vi "Make Channels Coincident.vi"(6 "interp. method":i32(ring) items=["nearest", "linear", "spline", "cubic Hermite", "Lagrange"], 8 "Time Cluster 2":T1, 9 "Time Cluster 1":T1, 10 "Cluster 2":T2={"Colour"=0, "Inst type"=enum."Pitot-static tube", "Inst name"="Manometer voltage", "Symbol"="U", "Code name"="", "Extra Info"="U", "Inst Array"=enum."PWA", "Extra Titles"=[], "Extra Values"=[], "U"=0.0, "u^2"=0.0, "u^3"=0.0, "u^4"=0.0, "Skew_u"=0.0, "Kurt_u"=0.0, "Sd Error in Mean"=0.0, "% u'/U"=0.0, "X"=0.0, "Y"=0.0, "Z"=0.0, "Timescale integral Estimate"=0.0, "Sd Error in Variance"=0.0, "Calib File"=path "", "Calib Constants"=[], "Output Position"=FALSE, "Stats"=enum."None", "Av Sampling Rate"=0.0, "Av No of Samples"=0.0, "Total Meas Time (s)"=0.0, "ADAM Ch Name"="", "Max value"=0.0, "Min value"=0.0, "Req Sample Rate Hz"=0.0, "Sync Delay Time (s)"=0.0, "Ch No"=0, "Device"="", "Use Latest Calib"=FALSE, "Port"="", "Metadata Ch Names"=[], "Metadata Ch Values"=[], "Label"=""} {"Sync Delay Time (s)" format="%.4f"; "Total Meas Time (s)" format="%_5g"; "Sd Error in Variance" format="%_3g"; "Skew_u" format="%_3g"; "% u'/U" format="%_3g"; "Sd Error in Mean" format="%_3g"; "Kurt_u" format="%_3g"; "u^4" format="%_3g"; "u^3" format="%_3g"; "U" format="%_3g"; "u^2" format="%_3g"}, 11 "Cluster 1":T2={"Colour"=0, "Inst type"=enum."Pitot-static tube", "Inst name"="Manometer voltage", "Symbol"="U", "Code name"="", "Extra Info"="U", "Inst Array"=enum."PWA", "Extra Titles"=[], "Extra Values"=[], "U"=0.0, "u^2"=0.0, "u^3"=0.0, "u^4"=0.0, "Skew_u"=0.0, "Kurt_u"=0.0, "Sd Error in Mean"=0.0, "% u'/U"=0.0, "X"=0.0, "Y"=0.0, "Z"=0.0, "Timescale integral Estimate"=0.0, "Sd Error in Variance"=0.0, "Calib File"=path "", "Calib Constants"=[], "Output Position"=FALSE, "Stats"=enum."None", "Av Sampling Rate"=0.0, "Av No of Samples"=0.0, "Total Meas Time (s)"=0.0, "ADAM Ch Name"="", "Max value"=0.0, "Min value"=0.0, "Req Sample Rate Hz"=0.0, "Sync Delay Time (s)"=0.0, "Ch No"=0, "Device"="", "Use Latest Calib"=FALSE, "Port"="", "Metadata Ch Names"=[], "Metadata Ch Values"=[], "Label"=""} {"Sync Delay Time (s)" format="%.4f"; "Total Meas Time (s)" format="%_5g"; "Sd Error in Variance" format="%_3g"; "Skew_u" format="%_3g"; "% u'/U" format="%_3g"; "Sd Error in Mean" format="%_3g"; "Kurt_u" format="%_3g"; "u^4" format="%_3g"; "u^3" format="%_3g"; "U" format="%_3g"; "u^2" format="%_3g"}) -> (0 "Time Window (ms)":dbl, 1 "Coincident Time Cluster 2":T1, 3 "Coincident Time Cluster 1":T1)   [LabVIEW 2021]
uses:
  Controls/Inst_type.ctl
  Controls/Instrument_Array.ctl
  Controls/Analysis_info_cluster.ctl
  Controls/Time_Trace_Cluster.ctl
panel:
  out "Time Window (ms) 2":dbl
  out "Array":i32[](array[numeric])
  out "Boolean":bool
  out "Frame":string
  in  "Show Plots":bool
  out "U1 and U2 Raw":cluster{"yi":dbl[], "yi":dbl[]}[](graph)
  out "U1 and U2 made coincident":cluster{"yi":dbl[], "yi":dbl[]}[](graph)
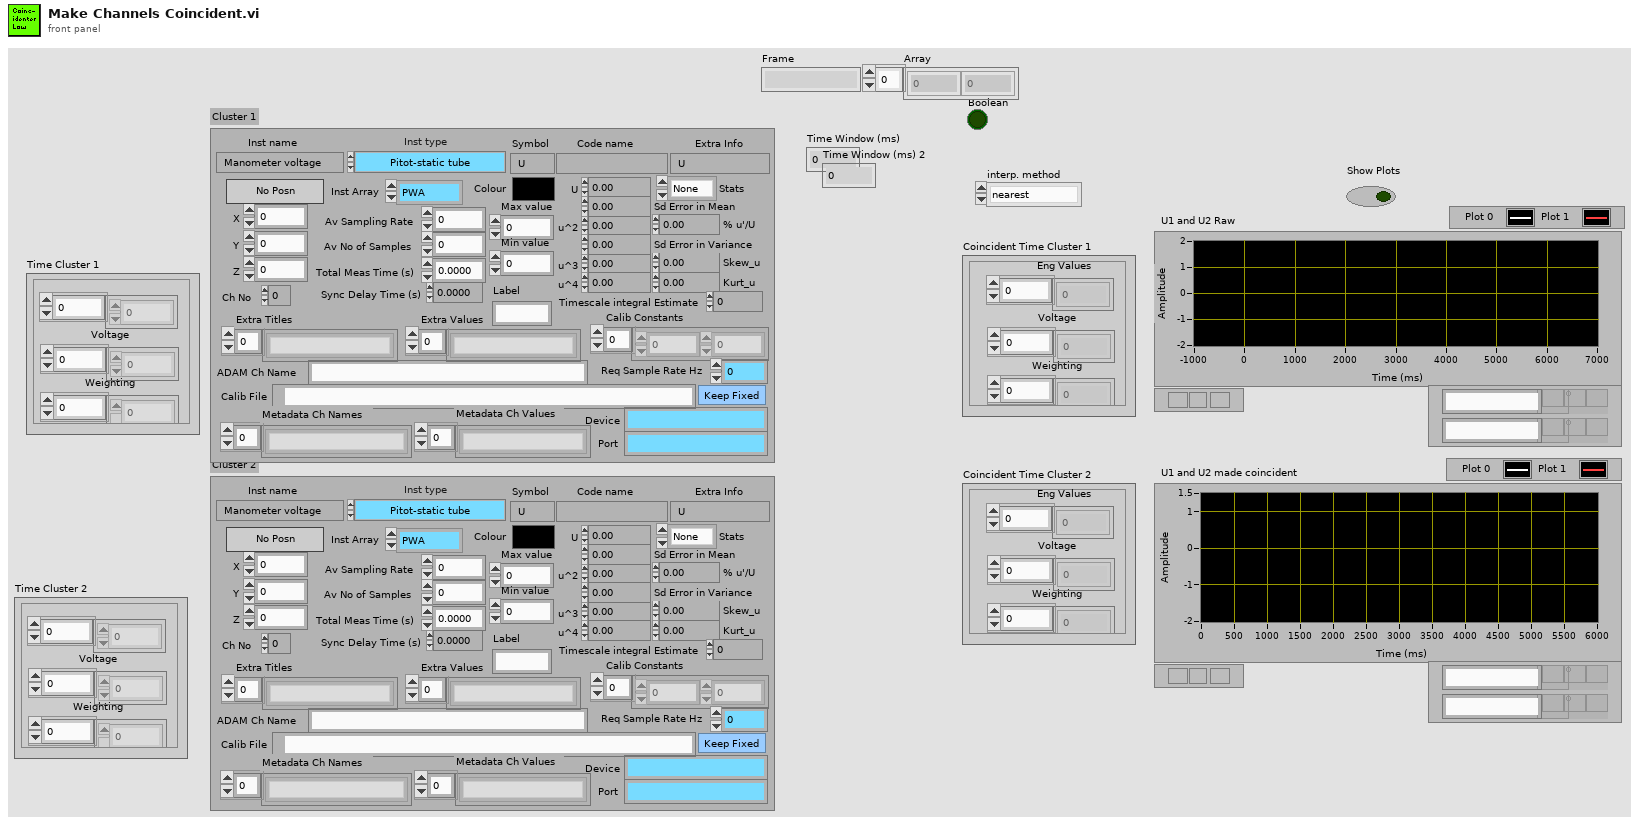
[diagram p1: front panel]
types:
  T1 = typedef "Time_Trace_Cluster.ctl" = cluster{"Weighting":dbl[], "Voltage":dbl[], "Eng Values":dbl[]}
  T2 = typedef "Analysis_info_cluster.ctl" = cluster{"Colour":u32, "Inst type":T3, "Inst name":string, "Symbol":string, "Code name":string, "Extra Info":string, "Inst Array":T4, "Extra Titles":string[], "Extra Values":string[], "U":dbl, "u^2":dbl, "u^3":dbl, "u^4":dbl, "Skew_u":dbl, "Kurt_u":dbl, "Sd Error in Mean":dbl, "% u'/U":dbl, "X":dbl, "Y":dbl, "Z":dbl, "Timescale integral Estimate":dbl, "Sd Error in Variance":dbl, "Calib File":path, "Calib Constants":dbl[], "Output Position":bool, "Stats":enum16{"None", "Basic", "Full"}, "Av Sampling Rate":dbl, "Av No of Samples":dbl, "Total Meas Time (s)":dbl, "ADAM Ch Name":string, "Max value":dbl, "Min value":dbl, "Req Sample Rate Hz":dbl, "Sync Delay Time (s)":dbl, "Ch No":i16, "Device":string, "Use Latest Calib":bool, "Port":string, "Metadata Ch Names":string[], "Metadata Ch Values":string[], "Label":string}
  T3 = typedef "Inst_type.ctl" = enum16{"Raw voltage", "Raw with zero offsetting", "Propeller anemometer", "Pressure Transducer", "Pitot-static tube", "Hot wire", "Cross wire 1", "Cross wire 2", "Generic Linear", "Generic Polynomial", "Generic BackPoly", "Fast FID", "Thermocouple", "Cold wire", "Pulsed Wire", "LDA Vel", "LDA Tran time", "LDA Arr time", "Microphone"}
  T4 = typedef "Instrument_Array.ctl" = enum16{"PWA", "LDA", "Analogue"}
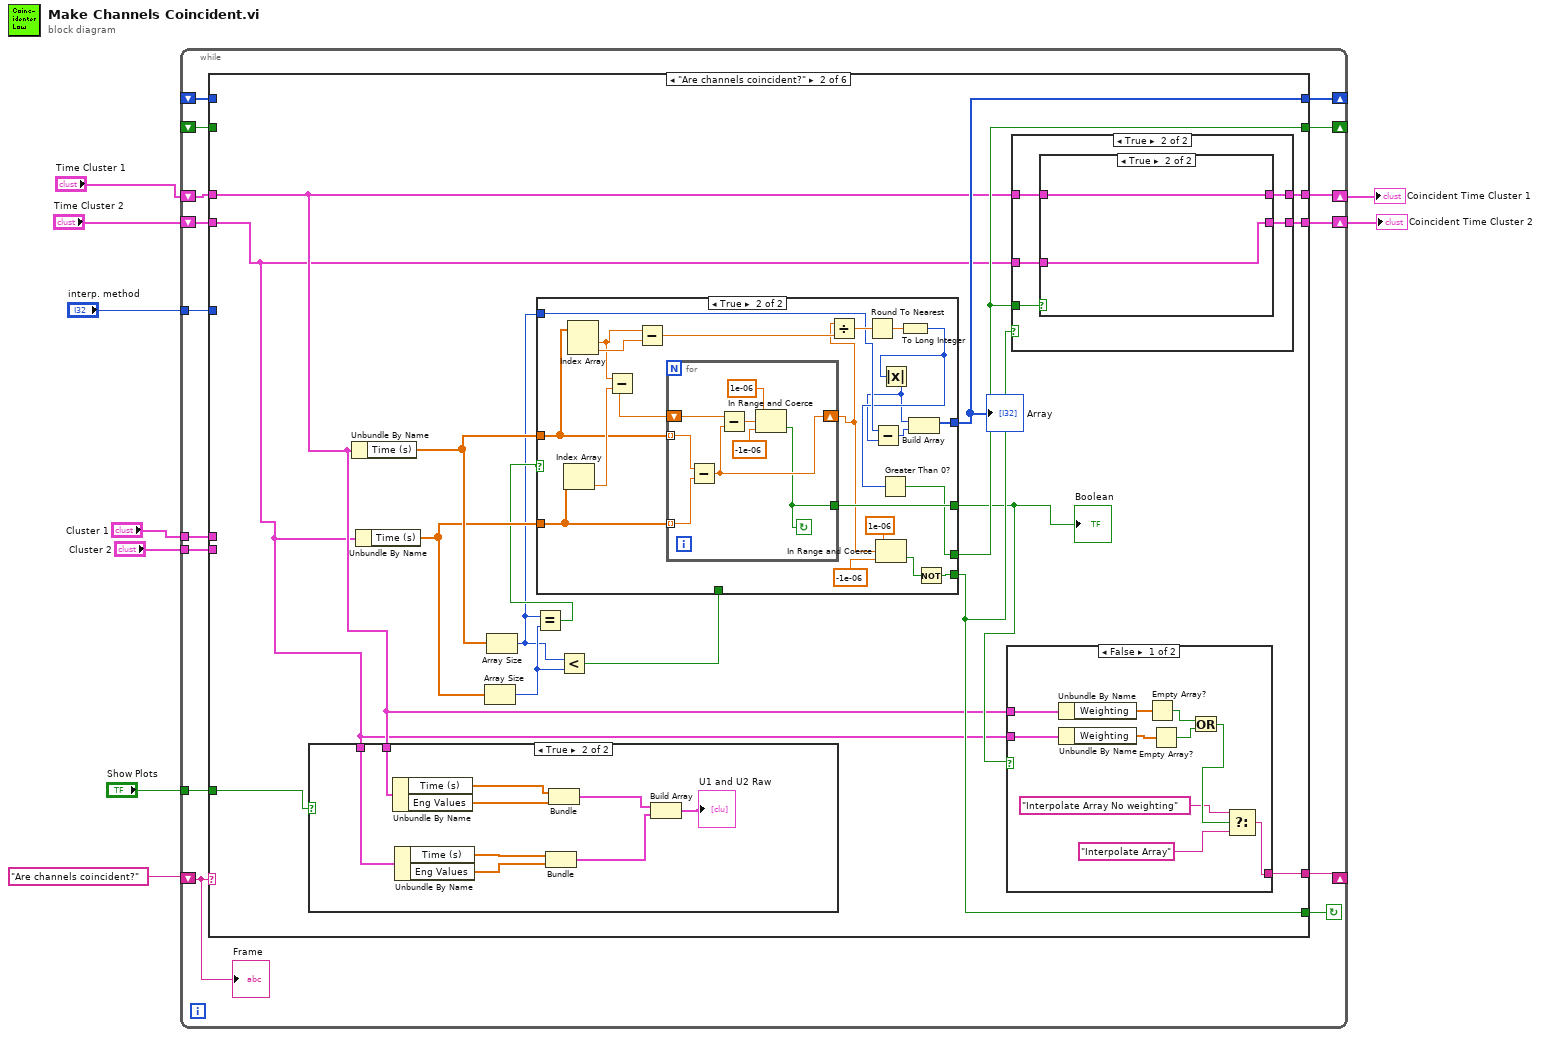
[diagram p0: block diagram]
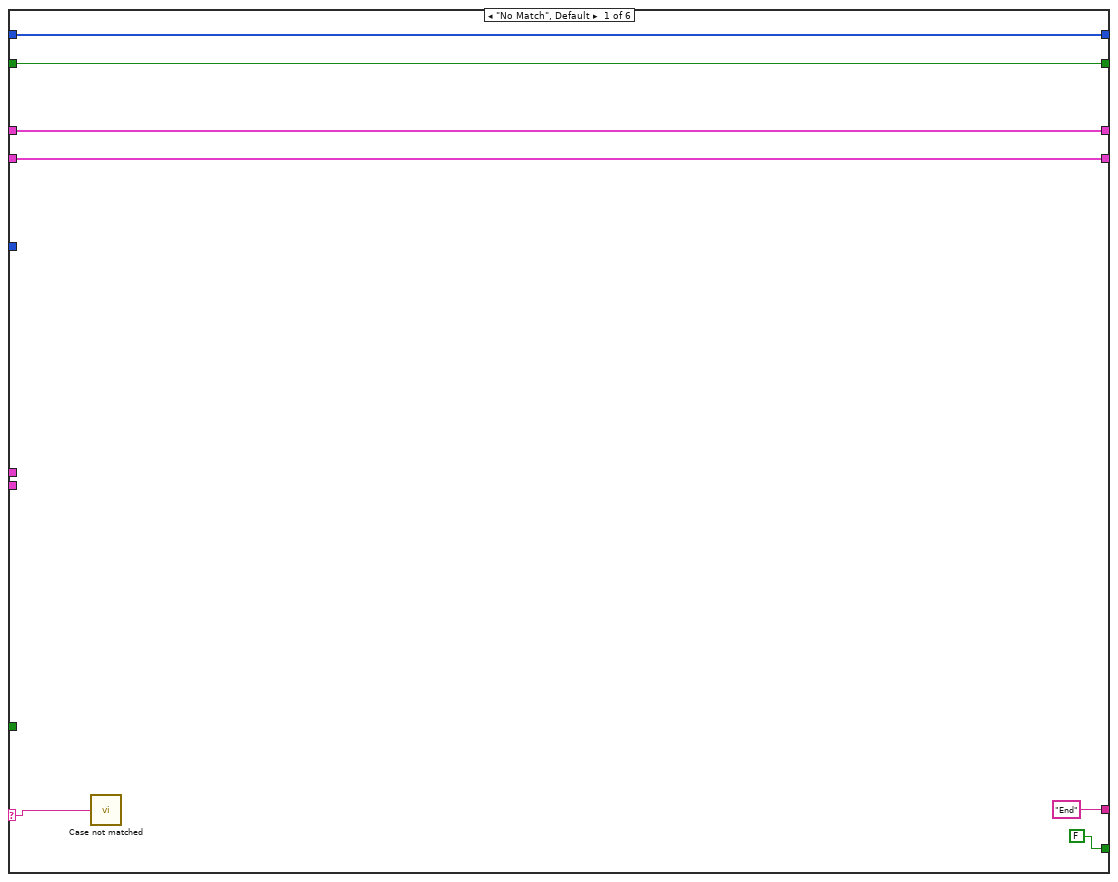
[diagram p2: hidden frame]
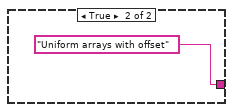
[diagram p3: hidden frame]
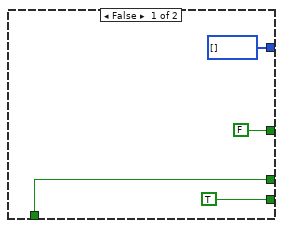
[diagram p4: hidden frame]
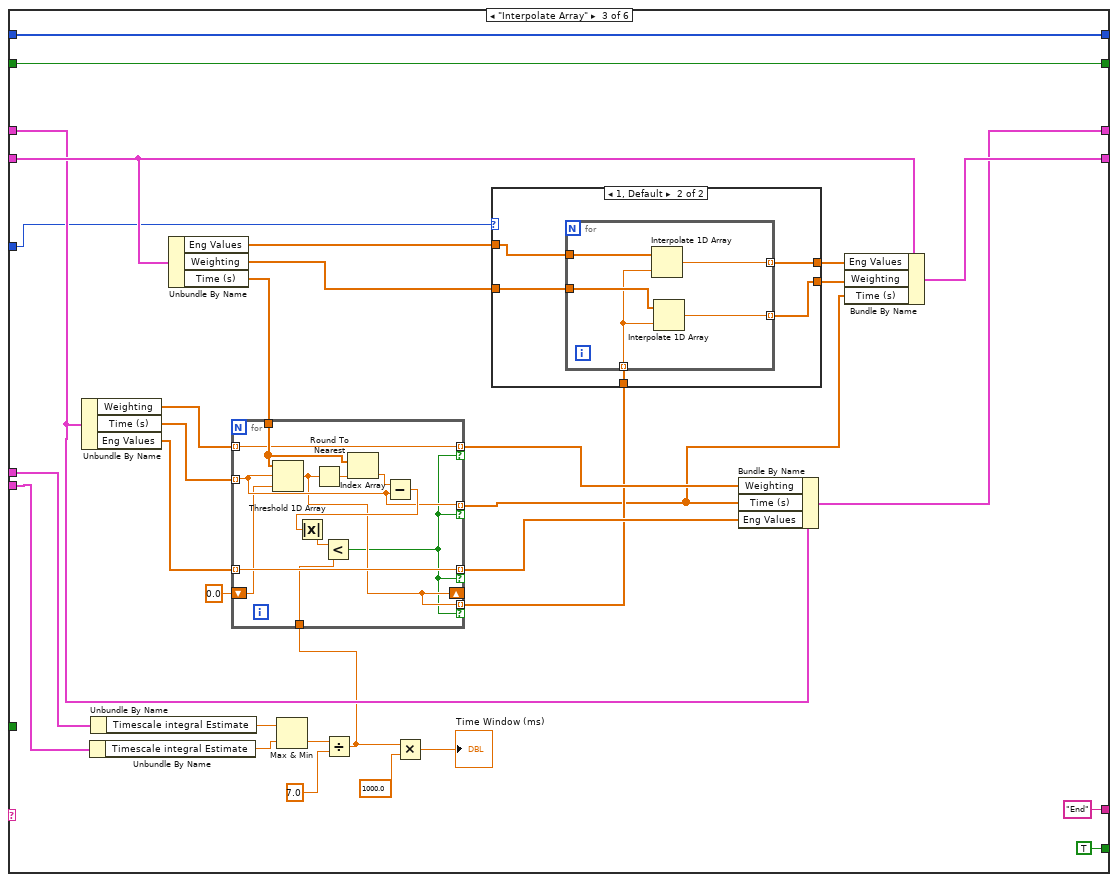
[diagram p8: hidden frame]
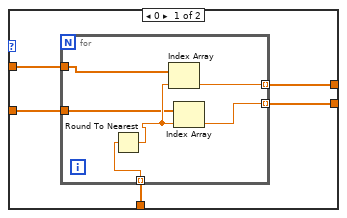
[diagram p9: hidden frame]
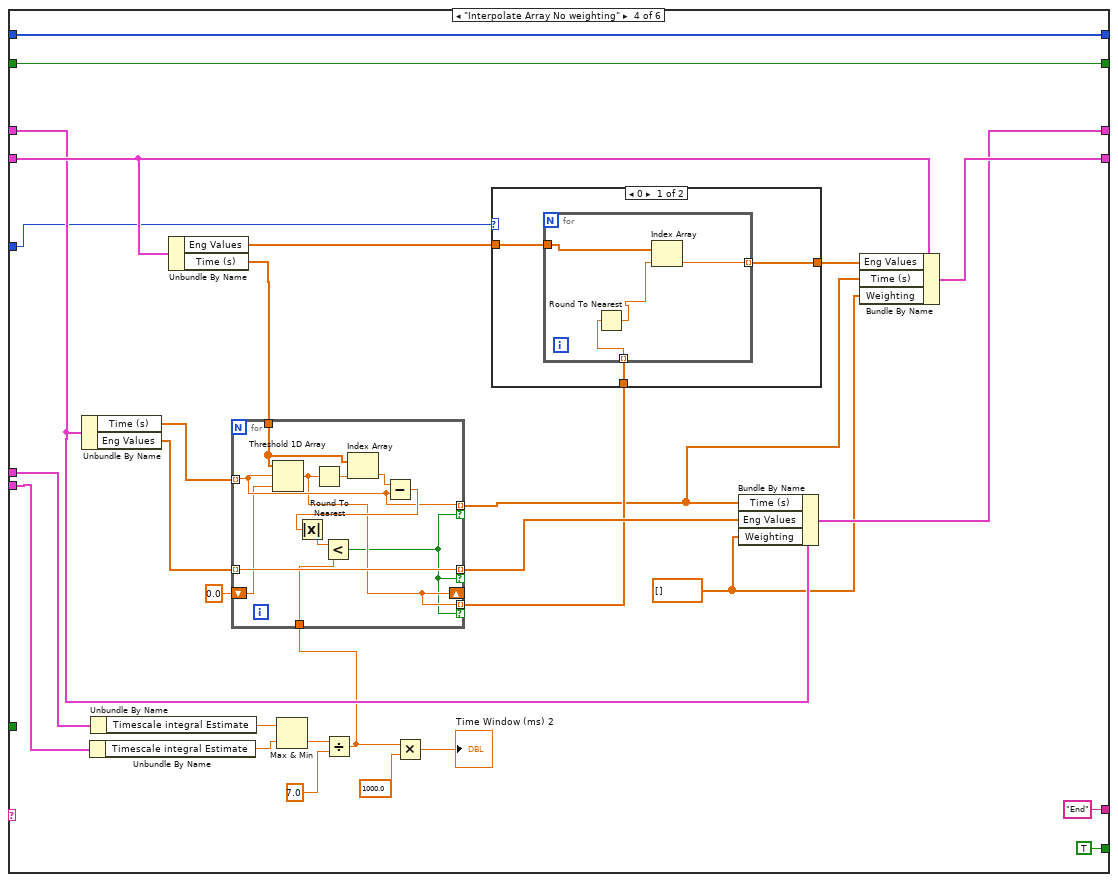
[diagram p10: hidden frame]
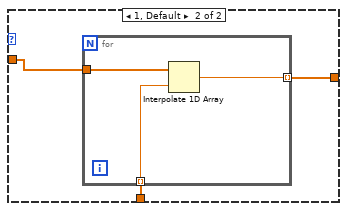
[diagram p11: hidden frame]
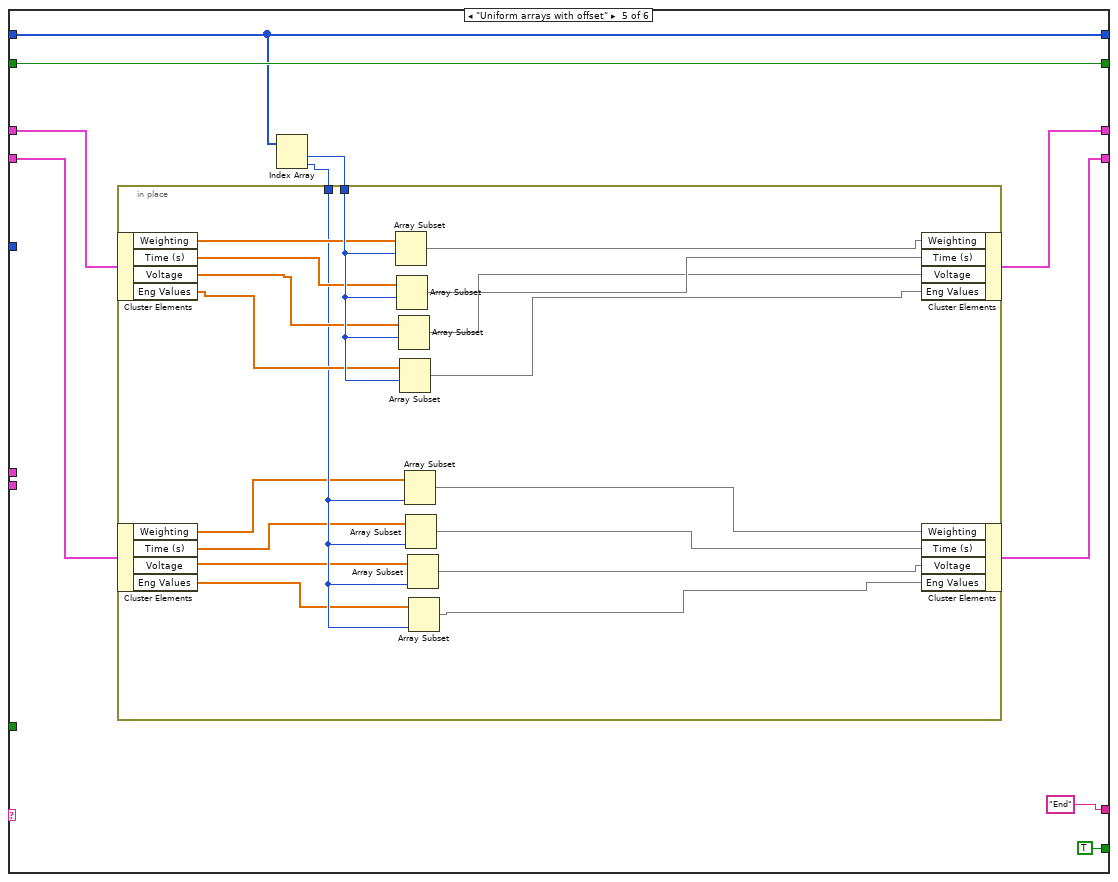
[diagram p12: hidden frame]
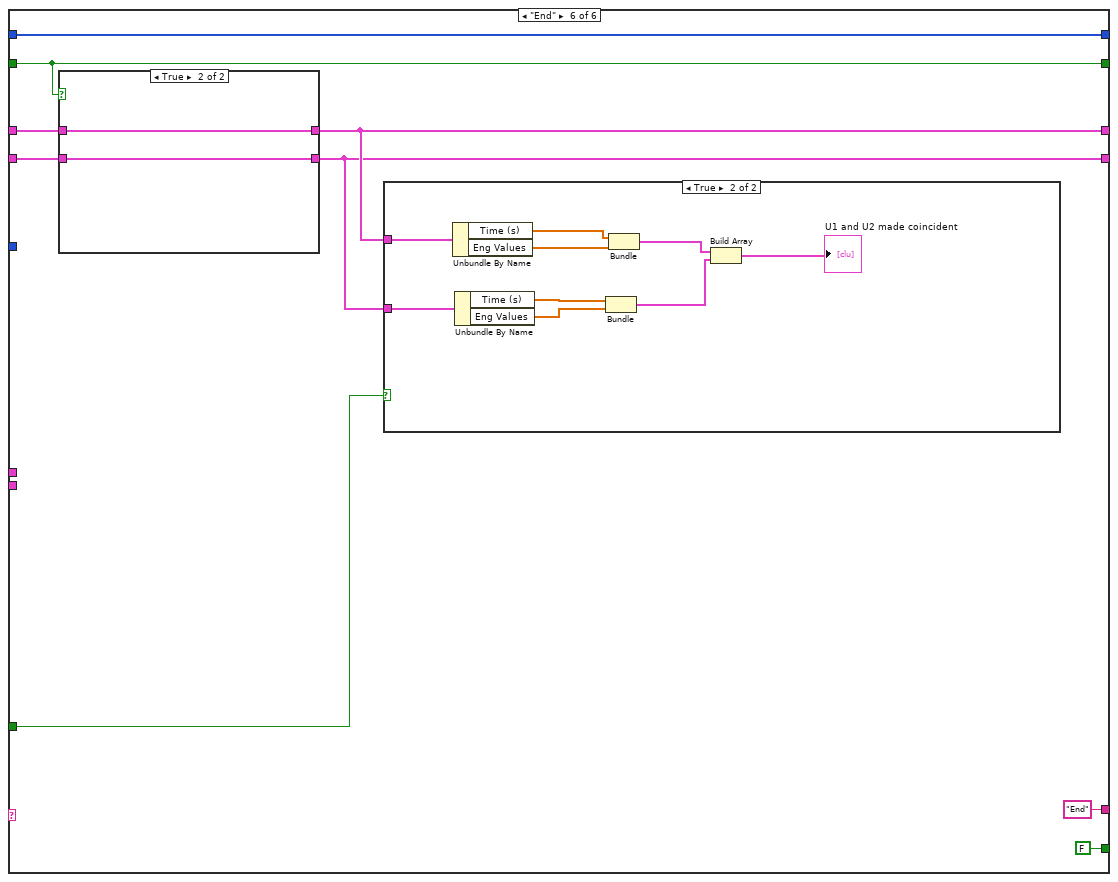
[diagram p13: hidden frame]
diagram:
  n1 = while {
    shift-right: [w19] -> w3
    shift-left: "Time Cluster 1" -> [w21]
    shift-right: [w18] -> w2
    shift-left: "Time Cluster 2" -> [w20]
    shift-right: [w22] -> _
    shift-left: "Are channels coincident?" -> [w24]
    tunnel: "Show Plots" -> [w17]
    tunnel: "Cluster 1" -> [w16]
    tunnel: "Cluster 2" -> [w15]
    shift-right: [w14] -> _
    shift-left: _ -> [w13]
    tunnel: "interp. method" -> [w12]
    shift-right: [w11] -> _
    shift-left: _ -> [w10]
    stop <- w23 continue-if-true
    n2 = case shown="\"Are channels coincident?\"" w24 {
      selector: w24 -> [w25 _ _ _ _ _]
      tunnel: [FALSE w36 TRUE TRUE TRUE FALSE] -> w23
      tunnel: ["End" w38 "End" "End" "End" "End" ("t")] -> w22
      tunnel: w21 -> [w29 w33 w134 w195 w237 w260]
      tunnel: w20 -> [w28 w32 w141 w202 w236 w258]
      tunnel: [w29 w46 w133 w194 w234 w261] -> w19
      tunnel: [w28 w47 w140 w201 w235 w259] -> w18
      tunnel: w17 -> [_ w45 _ _ _ w262]
      tunnel: w16 -> [_ _ w129 w193 _ _]
      tunnel: w15 -> [_ _ w128 w192 _ _]
      tunnel: [w27 w40 w138 w199 w233 w257] -> w14
      tunnel: w13 -> [w27 _ w138 w199 w233 w257]
      tunnel: w12 -> [_ _ w118 w182 _ _]
      tunnel: [w26 w37 w120 w184 w230 w256] -> w11
      tunnel: w10 -> [w26 _ w120 w184 w230 w256]
      frame "No Match", Default {
        n3 = call "Case not matched.vi"("Case Name not Matched"=w25) -> ()
      }
      frame "Are channels coincident?" {
        n4 = case shown="True" w45 {
          tunnel: w33 -> [_ w104]
          tunnel: w32 -> [_ w103]
          frame False {
          }
          frame True {
            n5 = Unbundle By Name(w104) -> ("Time (s)"=w105:dbl[], "Eng Values"=w109:dbl[])
            n6 = Unbundle By Name(w103) -> ("Time (s)"=w106:dbl[], "Eng Values"=w108:dbl[])
            n7 = Bundle("Time (s)"=w106, "Eng Values"=w108) -> (w107:cluster{"Time (s)":dbl[], "Eng Values":dbl[]})  [unwired: 1 in]
            n8 = Bundle("Time (s)"=w105, "Eng Values"=w109) -> (w110:cluster{"Time (s)":dbl[], "Eng Values":dbl[]})  [unwired: 1 in]
            n9 = Build Array(w110, w107) -> (→"U1 and U2 Raw":cluster{"Time (s)":dbl[], "Eng Values":dbl[]}[])
          }
        }
        n10 = Unbundle By Name(w33) -> ("Time (s)"=w44:dbl[])
        n11 = Unbundle By Name(w32) -> ("Time (s)"=w43:dbl[])
        n12 = Array Size(array=w43) -> (size(s)=w42:i32)
        n13 = Array Size(array=w44) -> (size(s)=w35:i32)
        n14 = Equal?(x=w35, y=w42) -> (x = y?=w41:bool)
        n15 = Less?(x=w35, y=w42) -> (x < y?=w39:bool)
        n16 = case shown="True" w41 {
          tunnel: w44 -> [_ w81]
          tunnel: w43 -> [_ w80]
          tunnel: [FALSE w79] -> w34
          tunnel: [i32[] [] w65] -> w37
          tunnel: [w61 w68] -> w40
          tunnel: w39 -> [w61 _]
          tunnel: [TRUE w76] -> w36
          tunnel: w35 -> [_ w66]
          frame False {
          }
          frame True {
            n17 = Index Array(array=w80) -> (element=w83:dbl)  [unwired: 1 in]
            n18 = Index Array(array=w81) -> (element #1=w73:dbl, element #2=w74:dbl)  [unwired: 2 in]
            n19 = Subtract(x=w73, y=w83) -> (x-y=w82:dbl)
            n20 = Subtract(x=w73, y=w74) -> (x-y=w71:dbl)
            n21 = for {
              tunnel: w81 -> [w91] mode=indexing
              tunnel: w80 -> [w90] mode=indexing
              shift-right: [w88] -> w70
              shift-left: w82 -> [w89]
              tunnel: [w84] -> w79
              stop <- w84 continue-if-true
              n22 = Subtract(x=w91, y=w90) -> (x-y=w88:dbl)
              n23 = Subtract(x=w89, y=w88) -> (x-y=w87:dbl)
              n24 = In Range and Coerce(upper limit=1e-06, x=w87, lower limit=-1e-06 ("upper limit")) -> (In Range?=w84:bool)  [unwired: 1 out]
            }
            n25 = Divide(x=w70, y=w71) -> (x/y=w72:dbl)
            n26 = Round To Nearest(number=w72) -> (nearest integer value=w69:dbl)
            n27 = In Range and Coerce(upper limit=1e-06, x=w70, lower limit=-1e-06 ("upper limit")) -> (In Range?=w75:bool)  [unwired: 1 out]
            n28 = To Long Integer(number=w69) -> (32bit integer=w64:i32)
            n29 = Greater Than 0?(x=w64) -> (x > 0?=w68:bool)
            n30 = Absolute Value(x=w64) -> (abs(x)=w63:i32)
            n31 = Subtract(x=w66, y=w63) -> (x-y=w67:i32)
            n32 = Build Array(w63, w67) -> (w65:i32[])
            n33 = Not(x=w75) -> (.not. x?=w76:bool)
          }
        }
        "Boolean" <- w34
        "Array" <- w37
        n34 = case shown="False" w34 {
          tunnel: [w49 "Uniform arrays with offset" ("t")] -> w38
          tunnel: w33 -> [w57 _]
          tunnel: w32 -> [w56 _]
          frame False {
            n35 = Unbundle By Name(w57) -> ("Weighting"=w55:dbl[])
            n36 = Unbundle By Name(w56) -> ("Weighting"=w54:dbl[])
            n37 = Empty Array?(array=w55) -> (empty?=w53:bool)
            n38 = Empty Array?(array=w54) -> (empty?=w52:bool)
            n39 = Or(x=w53, y=w52) -> (x .or. y?=w51:bool)
            n40 = Select(t="Interpolate Array No weighting", s=w51, f="Interpolate Array") -> (s? t:f=w49:string)
          }
          frame True {
          }
        }
        n41 = case shown="True" w36 {
          tunnel: [w92 w98] -> w47
          tunnel: [w93 w97] -> w46
          tunnel: w40 -> [_ w96]
          tunnel: w33 -> [w93 w95]
          tunnel: w32 -> [w92 w94]
          frame False {
          }
          frame True {
            n42 = case shown="True" w96 {
              tunnel: [w100 w101] -> w98
              tunnel: w95 -> [w100 w102]
              tunnel: w94 -> [w99 w101]
              tunnel: [w99 w102] -> w97
              frame False {
              }
              frame True {
              }
            }
          }
        }
      }
      frame "Interpolate Array" {
        n43 = Unbundle By Name(w134) -> ("Weighting"=w131:dbl[], "Time (s)"=w137:dbl[], "Eng Values"=w135:dbl[])
        n44 = Unbundle By Name(w128) -> ("Timescale integral Estimate"=w126:dbl)
        n45 = Unbundle By Name(w129) -> ("Timescale integral Estimate"=w127:dbl)
        n46 = Unbundle By Name(w141) -> ("Eng Values"=w117:dbl[], "Weighting"=w112:dbl[], "Time (s)"=w130:dbl[])
        n47 = Max & Min(x=w127, y=w126) -> (min(x,y)=w125:dbl)  [unwired: 1 out]
        n48 = Divide(x=w125, y=7.0) -> (x/y=w123:dbl)
        n49 = for {
          tunnel: w137 -> [w170] mode=indexing
          tunnel: w130 -> [w174]
          tunnel: [w170] -> w114 mode=indexing if=w164
          tunnel: [w169] -> w136 mode=indexing if=w164
          tunnel: w135 -> [w169] mode=indexing
          tunnel: [w168] -> w132 mode=indexing if=w164
          tunnel: w131 -> [w168] mode=indexing
          tunnel: w123 -> [w167]
          shift-right: [w165] -> _
          shift-left: 0.0 -> [w166]
          tunnel: [w165] -> w116 mode=indexing if=w164
          n50 = Threshold 1D Array(1:w166, 2:w170, 3:w174) -> (0:w165:dbl)
          n51 = Round To Nearest(number=w165) -> (nearest integer value=w175:dbl)
          n52 = Index Array(array=w174, index=w175) -> (element=w172:dbl)
          n53 = Subtract(x=w172, y=w170) -> (x-y=w171:dbl)
          n54 = Absolute Value(x=w171) -> (abs(x)=w173:dbl)
          n55 = Less?(x=w173, y=w167) -> (x < y?=w164:bool)
        }
        n56 = Multiply(x=w123, y=1000.0) -> (x*y=→"Time Window (ms)":dbl)
        n57 = case shown="1, Default" w118 {
          tunnel: w117 -> [w147 w157]
          tunnel: w116 -> [w146 w158]
          tunnel: [w145 w154] -> w115
          tunnel: [w144 w156] -> w113
          tunnel: w112 -> [w143 w155]
          frame 0 {
            n58 = for {
              tunnel: w147 -> [w151]
              tunnel: w146 -> [w153] mode=indexing
              tunnel: [w152] -> w145 mode=indexing
              tunnel: [w149] -> w144 mode=indexing
              tunnel: w143 -> [w148]
              n59 = Round To Nearest(number=w153) -> (nearest integer value=w150:dbl)
              n60 = Index Array(array=w151, index=w150) -> (element=w149:dbl)
              n61 = Index Array(array=w148, index=w150) -> (element=w152:dbl)
            }
          }
          frame 1, Default {
            n62 = for {
              tunnel: w158 -> [w160] mode=indexing
              tunnel: w157 -> [w163]
              tunnel: [w162] -> w156 mode=indexing
              tunnel: w155 -> [w161]
              tunnel: [w159] -> w154 mode=indexing
              n63 = Interpolate 1D Array(1:w160, 2:w163) -> (0:w162:dbl)
              n64 = Interpolate 1D Array(1:w160, 2:w161) -> (0:w159:dbl)
            }
          }
        }
        n65 = Bundle By Name(cluster=w134, "Weighting"=w132, "Time (s)"=w114, "Eng Values"=w136) -> (w133:T1)
        n66 = Bundle By Name(cluster=w141, "Eng Values"=w113, "Weighting"=w115, "Time (s)"=w114) -> (w140:T1)
      }
      frame "Interpolate Array No weighting" {
        w176 = dbl[] [] ("Weighting")
        n67 = Unbundle By Name(w195) -> ("Time (s)"=w198:dbl[], "Eng Values"=w196:dbl[])
        n68 = Unbundle By Name(w192) -> ("Timescale integral Estimate"=w190:dbl)
        n69 = Unbundle By Name(w193) -> ("Timescale integral Estimate"=w191:dbl)
        n70 = Unbundle By Name(w202) -> ("Eng Values"=w181:dbl[], "Time (s)"=w177:dbl[])
        n71 = Max & Min(x=w191, y=w190) -> (min(x,y)=w189:dbl)  [unwired: 1 out]
        n72 = Divide(x=w189, y=7.0) -> (x/y=w187:dbl)
        n73 = for {
          tunnel: w198 -> [w222] mode=indexing
          tunnel: w177 -> [w226]
          tunnel: [w222] -> w179 mode=indexing if=w217
          tunnel: [w221] -> w197 mode=indexing if=w217
          tunnel: w196 -> [w221] mode=indexing
          tunnel: w187 -> [w220]
          shift-right: [w218] -> _
          shift-left: 0.0 -> [w219]
          tunnel: [w218] -> w180 mode=indexing if=w217
          n74 = Threshold 1D Array(1:w219, 2:w222, 3:w226) -> (0:w218:dbl)
          n75 = Round To Nearest(number=w218) -> (nearest integer value=w227:dbl)
          n76 = Index Array(array=w226, index=w227) -> (element=w224:dbl)
          n77 = Subtract(x=w224, y=w222) -> (x-y=w223:dbl)
          n78 = Absolute Value(x=w223) -> (abs(x)=w225:dbl)
          n79 = Less?(x=w225, y=w220) -> (x < y?=w217:bool)
        }
        n80 = Multiply(x=w187, y=1000.0) -> (x*y=→"Time Window (ms) 2":dbl)
        n81 = case shown="0" w182 {
          tunnel: w181 -> [w206 w212]
          tunnel: w180 -> [w205 w213]
          tunnel: [w204 w211] -> w178
          frame 0 {
            n82 = for {
              tunnel: w206 -> [w209]
              tunnel: w205 -> [w210] mode=indexing
              tunnel: [w207] -> w204 mode=indexing
              n83 = Round To Nearest(number=w210) -> (nearest integer value=w208:dbl)
              n84 = Index Array(array=w209, index=w208) -> (element=w207:dbl)
            }
          }
          frame 1, Default {
            n85 = for {
              tunnel: w213 -> [w214] mode=indexing
              tunnel: w212 -> [w216]
              tunnel: [w215] -> w211 mode=indexing
              n86 = Interpolate 1D Array(1:w214, 2:w216) -> (0:w215:dbl)
            }
          }
        }
        n87 = Bundle By Name(cluster=w195, "Time (s)"=w179, "Eng Values"=w197, "Weighting"=w176) -> (w194:T1)
        n88 = Bundle By Name(cluster=w202, "Eng Values"=w178, "Time (s)"=w179, "Weighting"=w176) -> (w201:T1)
      }
      frame "Uniform arrays with offset" {
        n89 = Index Array(array=w230) -> (element #1=w229:i32, element #2=w228:i32)  [unwired: 2 in]
        n90 = in-place {
          in-place-border: w229 -> [w255]
          in-place-border: w228 -> [w246]
          n91 = in-place-cluster #1(w237) -> ("Weighting"=w254:dbl[], "Time (s)"=w253:dbl[], "Voltage"=w252:dbl[], "Eng Values"=w251:dbl[])
          n92 = in-place-cluster #2(w236) -> ("Weighting"=w245:dbl[], "Time (s)"=w244:dbl[], "Voltage"=w243:dbl[], "Eng Values"=w242:dbl[])
          n93 = Array Subset(array=w254, index=w255) -> (w250:dbl[])  [unwired: 1 in]
          n94 = Array Subset(array=w253, index=w255) -> (w249:dbl[])  [unwired: 1 in]
          n95 = Array Subset(array=w252, index=w255) -> (w248:dbl[])  [unwired: 1 in]
          n96 = Array Subset(array=w251, index=w255) -> (w247:dbl[])  [unwired: 1 in]
          n97 = Array Subset(array=w245, length=w246) -> (w241:dbl[])  [unwired: 1 in]
          n98 = Array Subset(array=w244, length=w246) -> (w240:dbl[])  [unwired: 1 in]
          n99 = Array Subset(array=w243, length=w246) -> (w239:dbl[])  [unwired: 1 in]
          n100 = Array Subset(array=w242, length=w246) -> (w238:dbl[])  [unwired: 1 in]
          n101 = in-place-cluster #1("Weighting"=w250, "Time (s)"=w249, "Voltage"=w248, "Eng Values"=w247) -> (w234:T1)
          n102 = in-place-cluster #2("Weighting"=w241, "Time (s)"=w240, "Voltage"=w239, "Eng Values"=w238) -> (w235:T1)
        }
      }
      frame "End" {
        n103 = case shown="True" w257 {
          tunnel: [w265 w268] -> w261
          tunnel: w260 -> [w266 w268]
          tunnel: [w266 w267] -> w259
          tunnel: w258 -> [w265 w267]
          frame False {
          }
          frame True {
          }
        }
        n104 = case shown="True" w262 {
          tunnel: w261 -> [_ w277]
          tunnel: w259 -> [_ w276]
          frame False {
          }
          frame True {
            n105 = Unbundle By Name(w277) -> ("Time (s)"=w270:dbl[], "Eng Values"=w274:dbl[])
            n106 = Unbundle By Name(w276) -> ("Time (s)"=w271:dbl[], "Eng Values"=w273:dbl[])
            n107 = Bundle("Time (s)"=w271, "Eng Values"=w273) -> (w272:cluster{"Time (s)":dbl[], "Eng Values":dbl[]})  [unwired: 1 in]
            n108 = Bundle("Time (s)"=w270, "Eng Values"=w274) -> (w275:cluster{"Time (s)":dbl[], "Eng Values":dbl[]})  [unwired: 1 in]
            n109 = Build Array(w275, w272) -> (→"U1 and U2 made coincident":cluster{"Time (s)":dbl[], "Eng Values":dbl[]}[])
          }
        }
      }
    }
    "Frame" <- w24
  }
  "Coincident Time Cluster 1" <- w3
  "Coincident Time Cluster 2" <- w2
